vi "PXI-Generate Test Pulse.vi"(0 "Line":tag, 7 "duration (ms)":dbl, 11 "error in (no error)":errorcluster) -> (15 "error out":errorcluster)   [LabVIEW 2020]
uses:
  <vilib>/DAQmx/write.llb/DAQmx Write (Digital Bool 1Line 1Point).vi
  <vilib>/DAQmx/create/channels.llb/DAQmx Create Channel (DO-Digital Output).vi
  <vilib>/DAQmx/miscellaneous.llb/DAQmx Fill In Error Info.vi
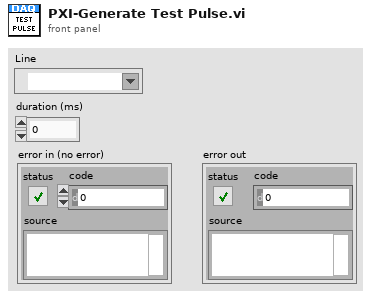
[diagram p1: front panel]
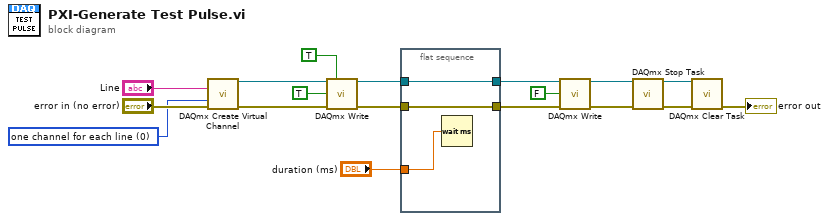
[diagram p0: block diagram]
diagram:
  w3 = 0 items=["one channel for each line", "one channel for all lines"] ("line grouping")
  n1 = call-poly <vilib>:"DAQmx Create Virtual Channel.vi"("lines"="Line", "line grouping"=w3, "error in"="error in (no error)") -> ("task out"=w4:refnum<k21>, "error out"=w6:errorcluster)  [unwired: 11 in]
  n2 = call-poly <vilib>:"DAQmx Write.vi"("task/channels in"=w4, "auto start"=TRUE, "data"=TRUE, "error in"=w6) -> ("task out"=w9:refnum<k21>, "error out"=w8:errorcluster)  [unwired: 9 in, 1 out]
  n3 = flat-sequence {
    tunnel: w8 -> [w21]
    tunnel: w9 -> [w20]
    tunnel: [w21] -> w11
    tunnel: [w20] -> w10
    tunnel: "duration (ms)" -> [w19]
    frame #0 {
      n4 = Wait (ms)(milliseconds to wait=w19) -> ()  [unwired: 1 out]
    }
  }
  n5 = call-poly <vilib>:"DAQmx Write.vi"("task/channels in"=w10, "data"=FALSE, "error in"=w11) -> ("task out"=w15:refnum<k21>, "error out"=w16:errorcluster)  [unwired: 10 in, 1 out]
  n6 = call <vilib>:"DAQmx Stop Task.vi"("task/channels in"=w15, "error in"=w16) -> ("task out"=w13:refnum<k21>, "error out"=w14:errorcluster)  [unwired: 12 in]
  n7 = call <vilib>:"DAQmx Clear Task.vi"("task in"=w13, "error in"=w14) -> ("error out"=→"error out":errorcluster)  [unwired: 13 in]
